vi "Read context in.vi"(8 "error in (no error)":errorcluster, 11 "Socket2 in":refnum<class "Socket2.lvclass">) -> (0 "error out":errorcluster, 2 "zeromq.lvlib:ZeroMQ Context":refnum<class "zmq_context.lvclass">, 3 "Socket2 out":refnum<class "Socket2.lvclass">)   [LabVIEW 2018, in "Socket2.lvclass"]
uses:
  Socket2.lvclass
  <vilib>/addons/zeromq/zmq_context.lvclass
  Socket2.lvclass/Socket2.ctl
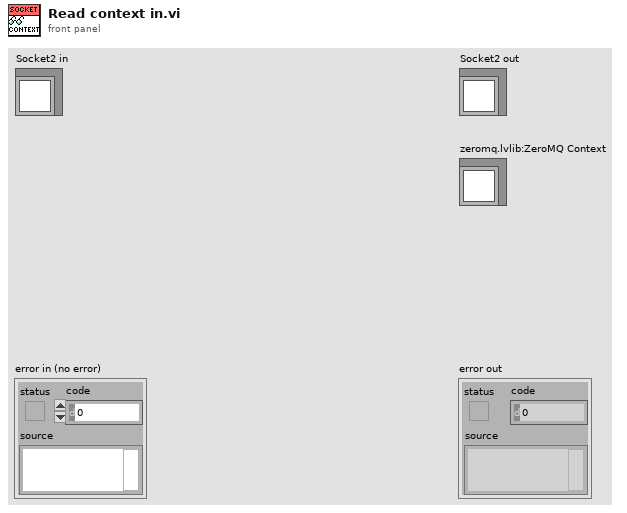
[diagram p1: front panel]
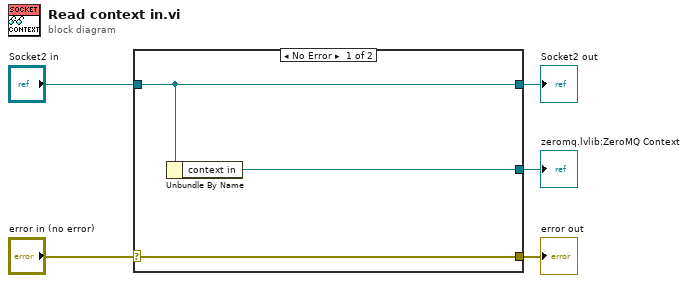
[diagram p0: block diagram]
diagram:
  n1 = case shown="No Error" "error in (no error)" {
    selector: "error in (no error)" -> [w8 w9]
    tunnel: [w8 w9] -> w4
    tunnel: [w7 w10] -> w2
    tunnel: "Socket2 in" -> [w7 w10]
    tunnel: [w6 _] -> w1
    frame No Error {
      n2 = Unbundle By Name(w7) -> ("context in"=w6:refnum<class "zmq_context.lvclass">)
    }
    frame Error {
    }
  }
  "error out" <- w4
  "Socket2 out" <- w2
  "zeromq.lvlib:ZeroMQ Context" <- w1
